vi "102-3102-report1p2-gaydos.vi"() -> ()   [LabVIEW 2012]
panel:
  out "Array 3":i32[](array[numeric])
  out "Array 2":string[](array[string])
  out "Waveform Graph":i8[](graph)
  in  "Numeric":dbl
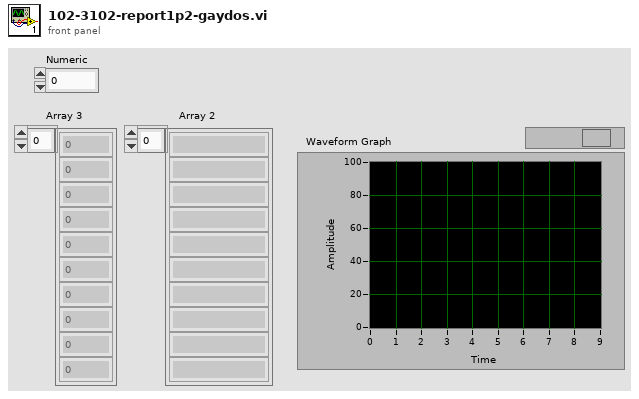
[diagram p1: front panel]
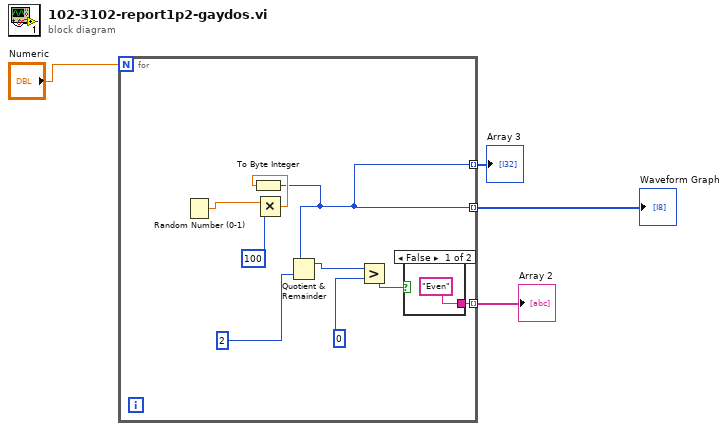
[diagram p0: block diagram]
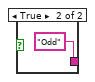
[diagram p2: hidden frame]
diagram:
  n1 = for {
    N: "Numeric" -> [_]
    tunnel: [w5] -> w3 mode=indexing
    tunnel: [w8] -> w2 mode=indexing
    tunnel: [w5] -> w1 mode=indexing
    n2 = Random Number (0-1)() -> (number: 0 to 1=w7:dbl)
    n3 = Multiply(x=w7, y=100) -> (x*y=w6:dbl)
    n4 = To Byte Integer(number=w6) -> (8bit integer=w5:i8)
    n5 = Quotient & Remainder(x=w5, y=2) -> (x-y*floor(x/y)=w10:i32)  [unwired: 1 out]
    n6 = Greater?(x=w10, y=0) -> (0:w9:bool)
    n7 = case shown="False" w9 {
      tunnel: ["Even" "Odd"] -> w8
      frame False {
      }
      frame True {
      }
    }
  }
  "Waveform Graph" <- w3
  "Array 2" <- w2
  "Array 3" <- w1
